vi "Get Array Size from Python String.vi"(11 "Python String":string) -> (1 "Array Size":i32, 3 "Python String out":string)   [LabVIEW 2020, in "jki_python_data_tools.lvlib"]
uses:
  jki_python_data_tools.lvlib
panel:
  # "Copyright © 2004-2009 JKI. All rights reserved.\n\nAuthor: Jim Kring [jim.kring@jameskring.com]\n\nThis library is provided \"AS IS\" ,WITHOUT WARRANTIES OR \nCONDITIONS OF ANY KIND, either express or implied.\n\nJames Kring, Inc. -- http://www.jameskring.com"
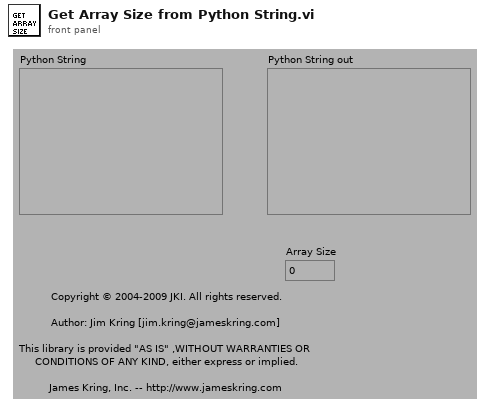
[diagram p1: front panel]
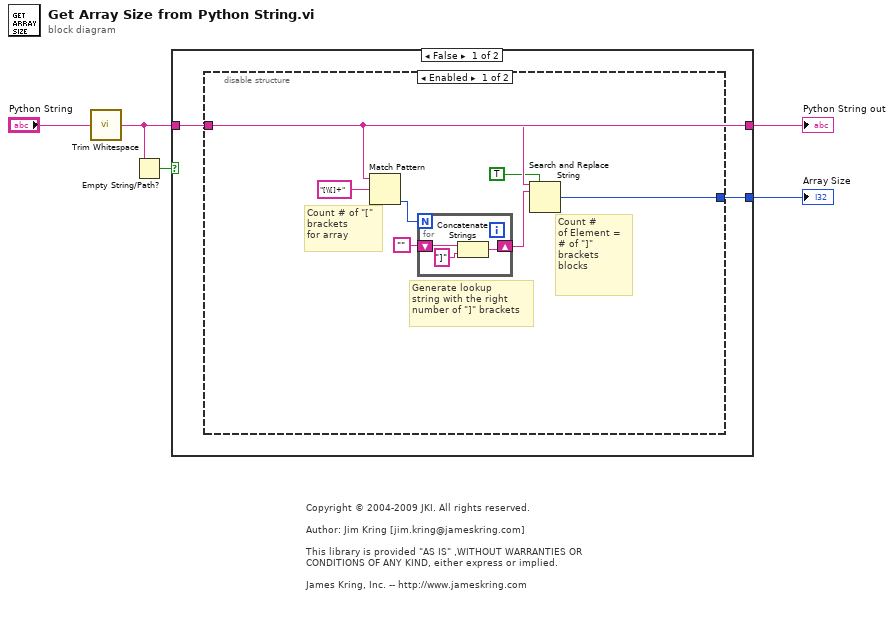
[diagram p0: block diagram]
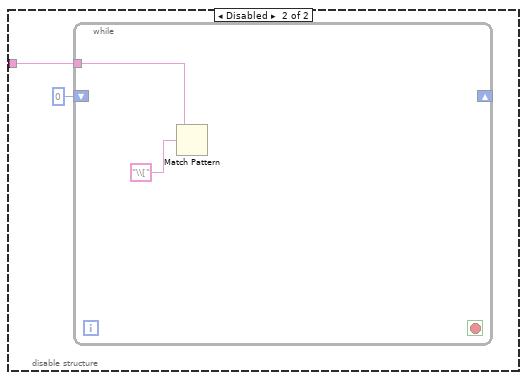
[diagram p2: hidden frame]
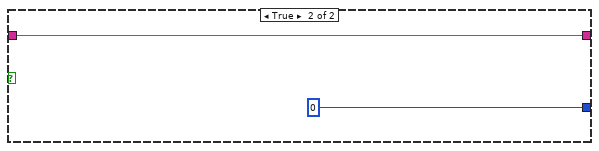
[diagram p3: hidden frame]
diagram:
  # "Copyright © 2004-2009 JKI. All rights reserved.\n\nAuthor: Jim Kring [jim.kring@jameskring.com]\n\nThis library is provided \"AS IS\" ,WITHOUT WARRANTIES OR \nCONDITIONS OF ANY KIND, either express or implied.\n\nJames Kring, Inc. -- http://www.jameskring.com"
  n1 = call <vilib>:"Trim Whitespace.vi"("string"="Python String") -> ("trimmed string"=w3:string)  [unwired: 1 in]
  n2 = Empty String/Path?(string/path=w3) -> (empty?=w2:bool)
  n3 = case shown="False" w2 {
    tunnel: [w7 0 ("number of replacements")] -> w5
    tunnel: w3 -> [w6 w23]
    tunnel: [w6 w23] -> w1
    frame False {
      n4 = disable-structure shown="Enabled" {
        disable-tunnel: [w14 _] -> w7
        disable-tunnel: w6 -> [w13 w19]
        frame Enabled {
          # "Generate lookup\nstring with the right\nnumber of \"]\" brackets"
          # "Count #\nof Element =\n# of \"]\" brackets blocks"
          # "Count # of \"[\"\nbrackets\nfor array"
          n5 = Match Pattern(string=w13, regular expression="[\\[]+") -> (offset past match=w10:i32)  [unwired: 1 in, 3 out]
          n6 = for {
            N: w10 -> [_]
            shift-right: [w15] -> w11
            shift-left: "" -> [w17]
            n7 = Concatenate Strings(w17, "]" ("regular expression")) -> (w15:string)
          }
          n8 = Search and Replace String(replace all?=TRUE ("replace all? (F)"), input string=w13, search string=w11) -> (number of replacements=w14:i32)  [unwired: 5 in, 3 out]
        }
        frame Disabled {
          n9 = while {
            shift-right: _ -> [_]
            shift-left: 0 -> [_]
            tunnel: w19 -> [w21]
            stop <- _ stop-if-true
            n10 = Match Pattern(string=w21, regular expression="\\[") -> ()  [unwired: 1 in, 4 out]
          }
        }
      }
    }
    frame True {
    }
  }
  "Array Size" <- w5
  "Python String out" <- w1
